vi "zlgcan_demo_USBCANFD_merge.vi"() -> ()   [LabVIEW 2020]
uses:
  zlgcan.lvlib
  data_type/ZCANDataObj.ctl
  data_type/ZCAN_InitCAN_setting_USBCANFD.ctl
  data_type/ZCAN_TransmitFD_frame.ctl
panel:
  in  "canfd_frame":T1
  in  "Clear Data":bool
  in  "stop":bool
  in  "开启CAN":bool
  in  "?":enum32{"DEMO说明", "设备、通道选择", "参数设置", "状态", "发送"}(tab)
  in  "CAN 通道":u32(ring) items=["0", "1"]
  in  "CAN卡型号":u32(ring)=41 items=["USBCANFD-800U"=59, "USBCANFD-200U"=41, "USBCANFD-100U"=42, "USBCANFD-MINI"=43]
  in  "索引":u32(ring) items=["0", "1", "2", "3", "4", "5", "6", "7", "8"]
  out "source":string
  in  "工作模式":u8(ring) items=["正常", "只听"]
  out "can_index_handle(out) 2":u32
  out "Device_handle(out)":u32
  out "can_index_handle(out)":u32
  in  "仲裁域波特率":u32(ring)=500000 items=["1Mbps"=1000000, "800kbps"=800000, "500kbps"=500000, "250kbps"=250000, "125kbps"=125000, "100kbps"=100000, "50kbps"=50000]
  in  "数据域波特率":u32(ring)=500000 items=["5Mbps"=5000000, "4Mbps"=4000000, "2Mbps"=2000000, "1Mbps"=1000000, "800kbps"=800000, "500kbps"=500000, "250kbps"=250000, "125kbps"=125000, "100kbps"=100000]
  in  "自定义波特率字符输入":string
  in  "自定义波特率开关":bool
  out "error out":errorcluster caption="错误输出"
  in  "数据长度":u8=8
  in  "CANFD accelerate":bool
  in  "Chennal":u32
  in  "帧类型":u32(ring) items=["标准帧", "扩展帧"]
  in  "帧格式":u32(ring) items=["数据帧", "远程帧"]
  in  "ID":u32=18 format="0x%08x"
  in  "协议":u32(ring) items=["CAN", "CANFD"]
  in  "数据输入":string="11 22 33 44 55 66 77 88"
  in  "发送":bool
  in  "timeStamp":u64=256
  out "Send Result":bool
  out "CAN报文显示":string[][](table)
  in  "ZCANDataObj":T2[](array[typedef])
  in  "ZCAN_InitCAN_Setting_USBCANFD":T3
  # "1. 确保电脑有VC++ 2005/2008/2010/2013运行库（对应32，64位）,微软常用运行库合集，点击下载（35M）。\n    http://manual.zlg.cn/Public/Uploads/2020-06-05/5ed995c271414.zip"
  # "2，如果打开设备失败，可能原因：\n（1）已经打开过一次，没有正常关闭的情况下，继续点击“打开设备”，是无法打开的。\n     需要USB重新拔插，LABVIEW重启（全部关闭），然后再“打开设备”。\n (2) 项目路径不能有中文繁体。"
  # "适用的设备：USBCANFD-100U、USBCANFD-200U、USBCANFD-MINI、USBCANFD-800U"
  # "停止程序前，\n请先关闭CAN卡"
  # "使用CAN时，\n两个波特率设置相同即可"
  # "使用ZCANPro软件波特率计算工具计算"
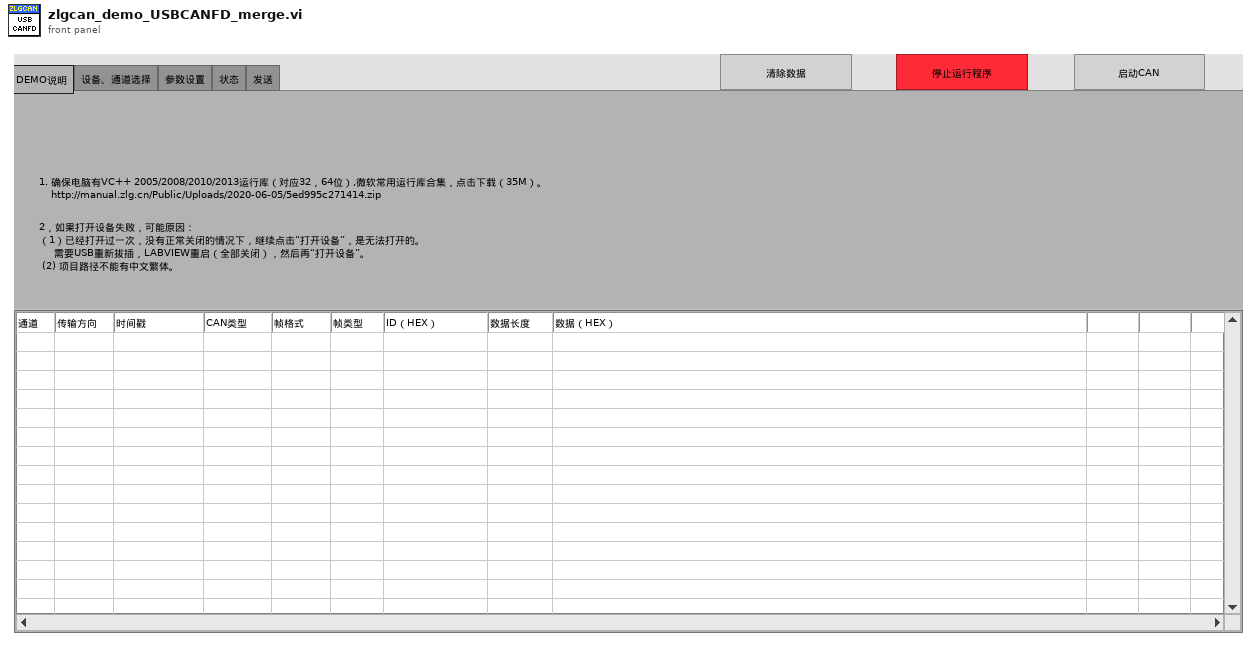
[diagram p1: front panel]
types:
  T1 = typedef "zlgcan.lvlib/ZCAN_TransmitFD_frame.ctl" = cluster{"帧类型":u32, "帧格式":u32, "ID":u32, "数据长度":u8, "CANFD加速？":u8, "DATA":cluster{"CAN数据[0]":u8, "CAN数据[1]":u8, "CAN数据[2]":u8, "CAN数据[3]":u8, "CAN数据[4]":u8, "CAN数据[5]":u8, "CAN数据[6]":u8, "CAN数据[7]":u8, "CAN数据[8]":u8, "CAN数据[9]":u8, "CAN数据[10]":u8, "CAN数据[11] ":u8, "CAN数据[12] ":u8, "CAN数据[13] ":u8, "CAN数据[14] ":u8, "CAN数据[15] ":u8, "CAN数据[16]":u8, "CAN数据[17]":u8, "CAN数据[18]":u8, "CAN数据[19]":u8, "CAN数据[20]":u8, "CAN数据[21]":u8, "CAN数据[22]":u8, "CAN数据[23]":u8, "CAN数据[24] ":u8, "CAN数据[25]":u8, "CAN数据[26]":u8, "CAN数据[27]":u8, "CAN数据[28]":u8, "CAN数据[29]":u8, "CAN数据[30]":u8, "CAN数据[31]":u8, "CAN数据[32]":u8, "CAN数据[33]":u8, "CAN数据[34]":u8, "CAN数据[35]":u8, "CAN数据[36]":u8, "CAN数据[37]":u8, "CAN数据[38]":u8, "CAN数据[39]":u8, "CAN数据[40]":u8, "CAN数据[41]":u8, "CAN数据[42]":u8, "CAN数据[43]":u8, "CAN数据[44]":u8, "CAN数据[45]":u8, "CAN数据[46]":u8, "CAN数据[47]":u8, "CAN数据[48]":u8, "CAN数据[49]":u8, "CAN数据[50]":u8, "CAN数据[51]":u8, "CAN数据[52]":u8, "CAN数据[53]":u8, "CAN数据[54]":u8, "CAN数据[55]":u8, "CAN数据[56]":u8, "CAN数据[57]":u8, "CAN数据[58]":u8, "CAN数据[59]":u8, "CAN数据[60]":u8, "CAN数据[61]":u8, "CAN数据[62]":u8, "CAN数据[63]":u8}}
  T2 = typedef "zlgcan.lvlib/ZCANDataObj.ctl" = cluster{"Data_Type":u8, "CAN_CH":u8, "rawVal(未使用)":u16, "extraData[4]（未使用）":cluster{"[0]":u8, "[1]":u8, "[2]":u8, "[3]":u8}, "canCANFDData":cluster{"时间戳+混合标志位":cluster{"时间戳":u64, "混合标志位":u32}, "extraData[4]（未使用）":cluster{"[0]":u8, "[1]":u8, "[2]":u8, "[3]":u8}, "frame":cluster{"can_id":u32, "Data长度":u8, "CANFD加速？":u8, "__res0":u8, "__res1":u8, "data":cluster{"CANData[0]":u8, "CANData[1]":u8, "CANData[2]":u8, "CANData[3]":u8, "CANData[4]":u8, "CANData[5]":u8, "CANData[6]":u8, "CANData[7]":u8, "CANData[8]":u8, "CANData[9]":u8, "CANData[10]":u8, "CANData[11] ":u8, "CANData[12] ":u8, "CANData[13] ":u8, "CANData[14] ":u8, "CANData[15] ":u8, "CANData[16]":u8, "CANData[17]":u8, "CANData[18]":u8, "CANData[19]":u8, "CANData[20]":u8, "CANData[21]":u8, "CANData[22]":u8, "CANData[23]":u8, "CANData[24] ":u8, "CANData[25]":u8, "CANData[26]":u8, "CANData[27]":u8, "CANData[28]":u8, "CANData[29]":u8, "CANData[30]":u8, "CANData[31]":u8, "CANData[32]":u8, "CANData[33]":u8, "CANData[34]":u8, "CANData[35]":u8, "CANData[36]":u8, "CANData[37]":u8, "CANData[38]":u8, "CANData[39]":u8, "CANData[40]":u8, "CANData[41]":u8, "CANData[42]":u8, "CANData[43]":u8, "CANData[44]":u8, "CANData[45]":u8, "CANData[46]":u8, "CANData[47]":u8, "CANData[48]":u8, "CANData[49]":u8, "CANData[50]":u8, "CANData[51]":u8, "CANData[52]":u8, "CANData[53]":u8, "CANData[54]":u8, "CANData[55]":u8, "CANData[56]":u8, "CANData[57]":u8, "CANData[58]":u8, "CANData[59]":u8, "CANData[60]":u8, "CANData[61]":u8, "CANData[62]":u8, "CANData[63]":u8}}}, "raw":cluster{"[0]":u8, "[1]":u8, "[2]":u8, "[3]":u8, "[4]":u8, "[5]":u8, "[6]":u8, "[7]":u8, "[8]":u8, "[9]":u8, "[10]":u8, "[11]":u8, "[12]":u8, "[13]":u8, "[14]":u8, "[15]":u8, "[16]":u8, "[17]":u8, "[18]":u8, "[19]":u8, "[20]":u8, "[21]":u8, "[22]":u8, "[23]":u8, "[24]":u8, "[25]":u8, "[26]":u8, "[27]":u8, "[28]":u8, "[29]":u8, "[30]":u8, "[31]":u8, "[32]":u8, "[33]":u8, "[34]":u8, "[35]":u8, "[36]":u8, "[37]":u8, "[38]":u8, "[39]":u8, "[40]":u8, "[41]":u8, "[42]":u8, "[43]":u8, "[44]":u8, "[45]":u8, "[46]":u8, "[47]":u8, "[48]":u8, "[49]":u8, "[50]":u8, "[51]":u8, "[52]":u8, "[53]":u8, "[54]":u8, "[55]":u8, "[56]":u8, "[57]":u8, "[58]":u8, "[59]":u8, "[60]":u8, "[61]":u8, "[62]":u8, "[63]":u8, "[64]":u8, "[65]":u8, "[73]":u8, "[72]":u8, "[71]":u8, "[70]":u8, "[69]":u8, "[68]":u8, "[67]":u8, "[66]":u8, "[74]":u8, "[75]":u8, "[83]":u8, "[82]":u8, "[81]":u8, "[80]":u8, "[79]":u8, "[78]":u8, "[77]":u8, "[76]":u8, "[84]":u8, "[85]":u8, "[91]":u8, "[90]":u8, "[89]":u8, "[88]":u8, "[87]":u8, "[86]":u8}}
  T3 = typedef "zlgcan.lvlib/ZCAN_InitCAN_setting_USBCANFD.ctl" = cluster{"abitbaud":u32, "dbitbaud":u32, "baud_rate_custom？":bool, "RateCustom":string, "mode":u8}
  T4 = cluster{"[0]":u32, "[1]":u32, "[2]":u32, "[3]":u32, "[4]":u32, "[5]":u32, "[6]":u32, "[7]":u32, "[8]":u32, "[9]":u32, "[10]":u32, "[11]":u32, "[12]":u32, "[13]":u32, "[14]":u32, "[15]":u32, "[16]":u32, "[17]":u32, "[18]":u32, "[19]":u32, "[20]":u32, "[21]":u32, "[22]":u32, "[23]":u32, "[24]":u32, "[25]":u32, "[26]":u32, "[27]":u32, "[28]":u32, "[29]":u32, "[30]":u32, "[31]":u32, "[32]":u32, "[33]":u32, "[34]":u32, "[35]":u32, "[36]":u32, "[37]":u32, "[38]":u32, "[39]":u32, "[40]":u32, "[41]":u32, "[42]":u32, "[43]":u32, "[44]":u32, "[45]":u32, "[46]":u32, "[47]":u32, "[48]":u32, "[49]":u32, "[50]":u32, "[51]":u32, "[52]":u32, "[53]":u32, "[54]":u32, "[55]":u32, "[56]":u32, "[57]":u32, "[58]":u32, "[59]":u32, "[60]":u32, "[61]":u32, "[62]":u32, "[63]":u32}
  T5 = typedef "ZCANDataObj.ctl" = cluster{"数据类型":u8, "CAN通道号":u8, "rawVal(未使用)":u16, "extraData[4]（未使用）":cluster{"[0]":u8, "[1]":u8, "[2]":u8, "[3]":u8}, "canCANFDData":cluster{"时间戳+混合标志位":cluster{"时间戳":u64, "混合标志位":u32}, "extraData[4]（未使用）":cluster{"[0]":u8, "[1]":u8, "[2]":u8, "[3]":u8}, "frame":cluster{"can_id":u32, "数据长度":u8, "CANFD加速？":u8, "__res0":u8, "__res1":u8, "data":cluster{"CAN数据[0]":u8, "CAN数据[1]":u8, "CAN数据[2]":u8, "CAN数据[3]":u8, "CAN数据[4]":u8, "CAN数据[5]":u8, "CAN数据[6]":u8, "CAN数据[7]":u8, "CAN数据[8]":u8, "CAN数据[9]":u8, "CAN数据[10]":u8, "CAN数据[11] ":u8, "CAN数据[12] ":u8, "CAN数据[13] ":u8, "CAN数据[14] ":u8, "CAN数据[15] ":u8, "CAN数据[16]":u8, "CAN数据[17]":u8, "CAN数据[18]":u8, "CAN数据[19]":u8, "CAN数据[20]":u8, "CAN数据[21]":u8, "CAN数据[22]":u8, "CAN数据[23]":u8, "CAN数据[24] ":u8, "CAN数据[25]":u8, "CAN数据[26]":u8, "CAN数据[27]":u8, "CAN数据[28]":u8, "CAN数据[29]":u8, "CAN数据[30]":u8, "CAN数据[31]":u8, "CAN数据[32]":u8, "CAN数据[33]":u8, "CAN数据[34]":u8, "CAN数据[35]":u8, "CAN数据[36]":u8, "CAN数据[37]":u8, "CAN数据[38]":u8, "CAN数据[39]":u8, "CAN数据[40]":u8, "CAN数据[41]":u8, "CAN数据[42]":u8, "CAN数据[43]":u8, "CAN数据[44]":u8, "CAN数据[45]":u8, "CAN数据[46]":u8, "CAN数据[47]":u8, "CAN数据[48]":u8, "CAN数据[49]":u8, "CAN数据[50]":u8, "CAN数据[51]":u8, "CAN数据[52]":u8, "CAN数据[53]":u8, "CAN数据[54]":u8, "CAN数据[55]":u8, "CAN数据[56]":u8, "CAN数据[57]":u8, "CAN数据[58]":u8, "CAN数据[59]":u8, "CAN数据[60]":u8, "CAN数据[61]":u8, "CAN数据[62]":u8, "CAN数据[63]":u8}}}, "Reserve":u32}
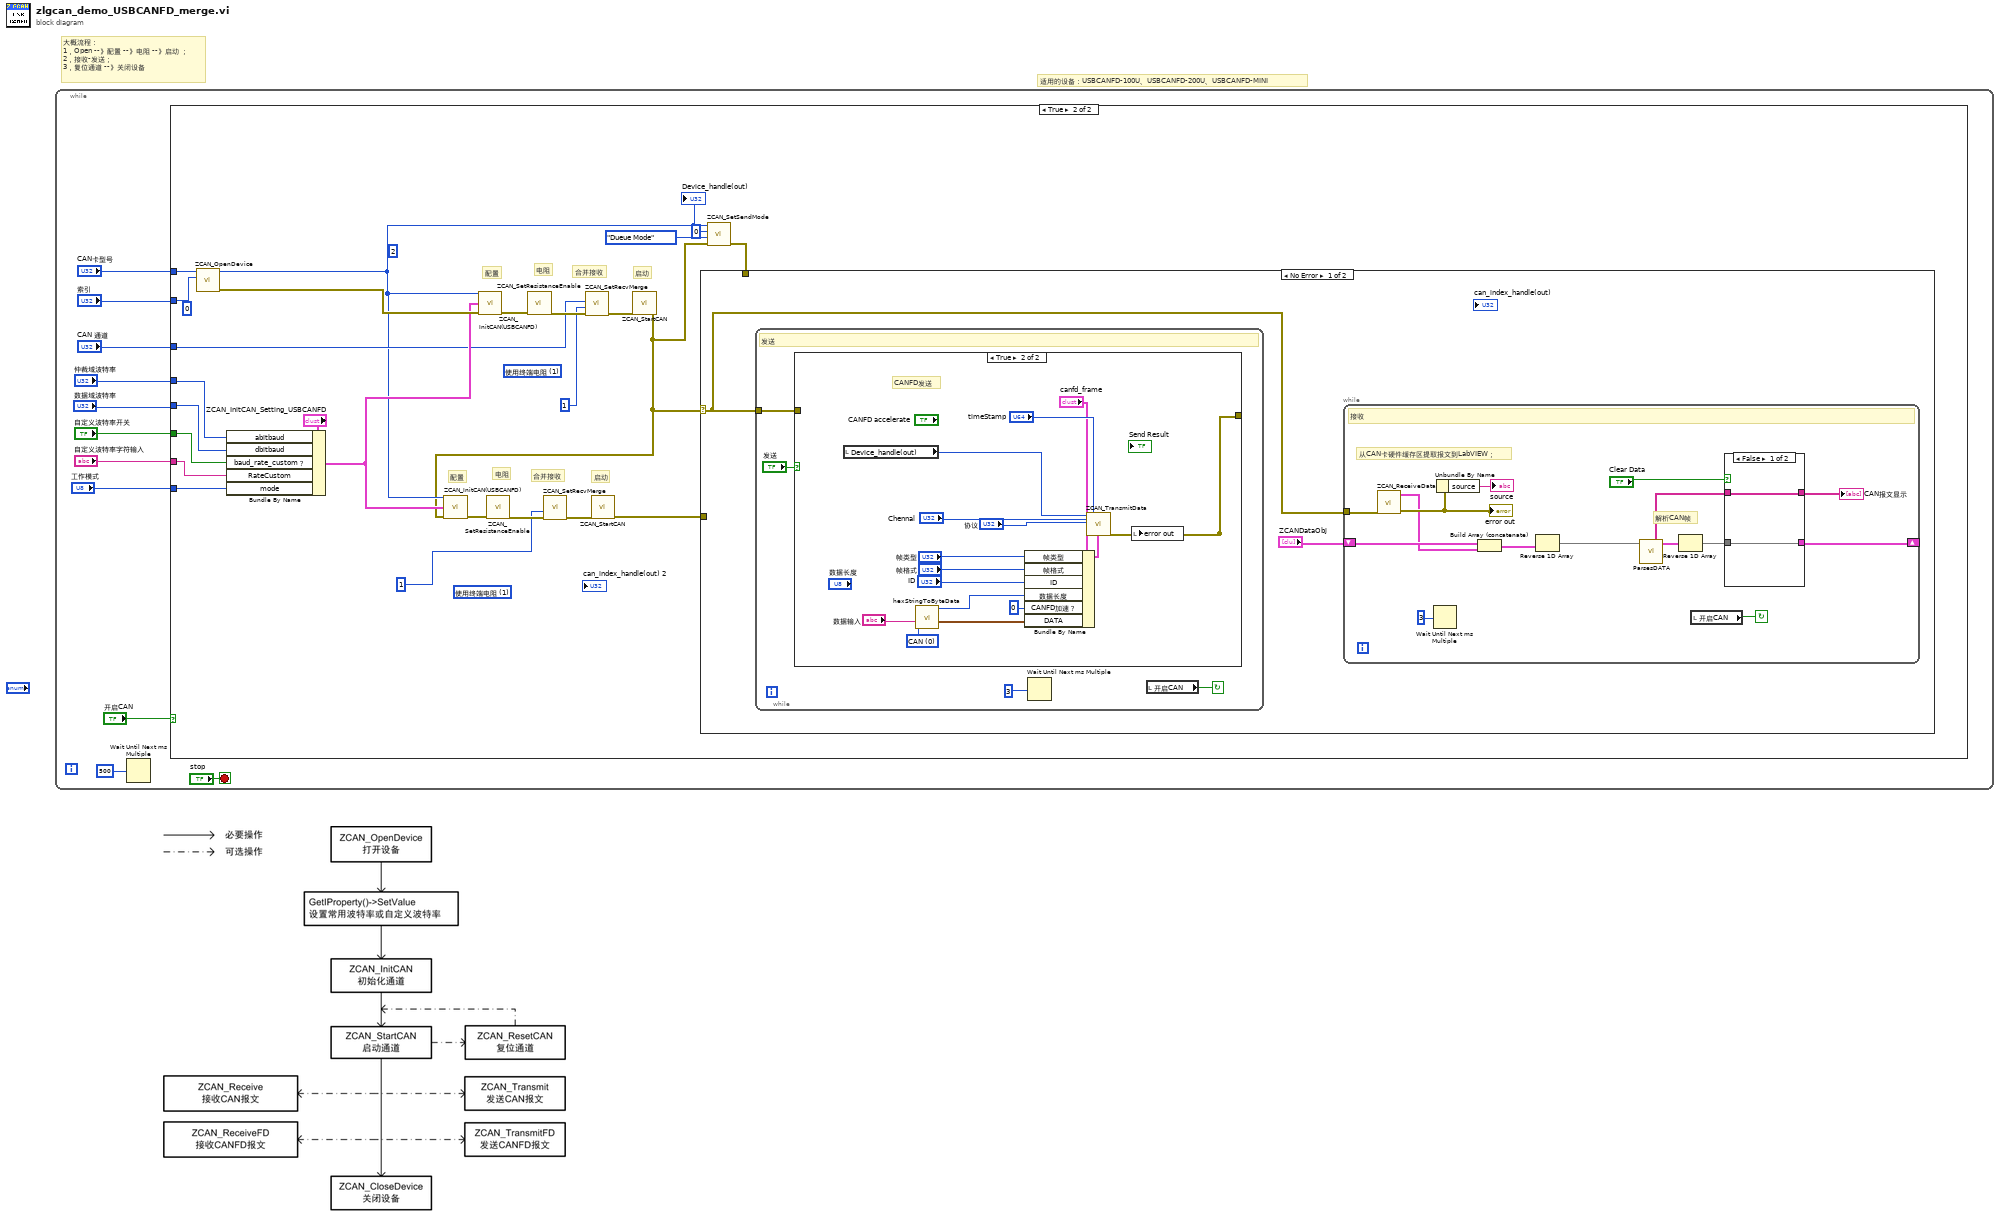
[diagram p0: block diagram]
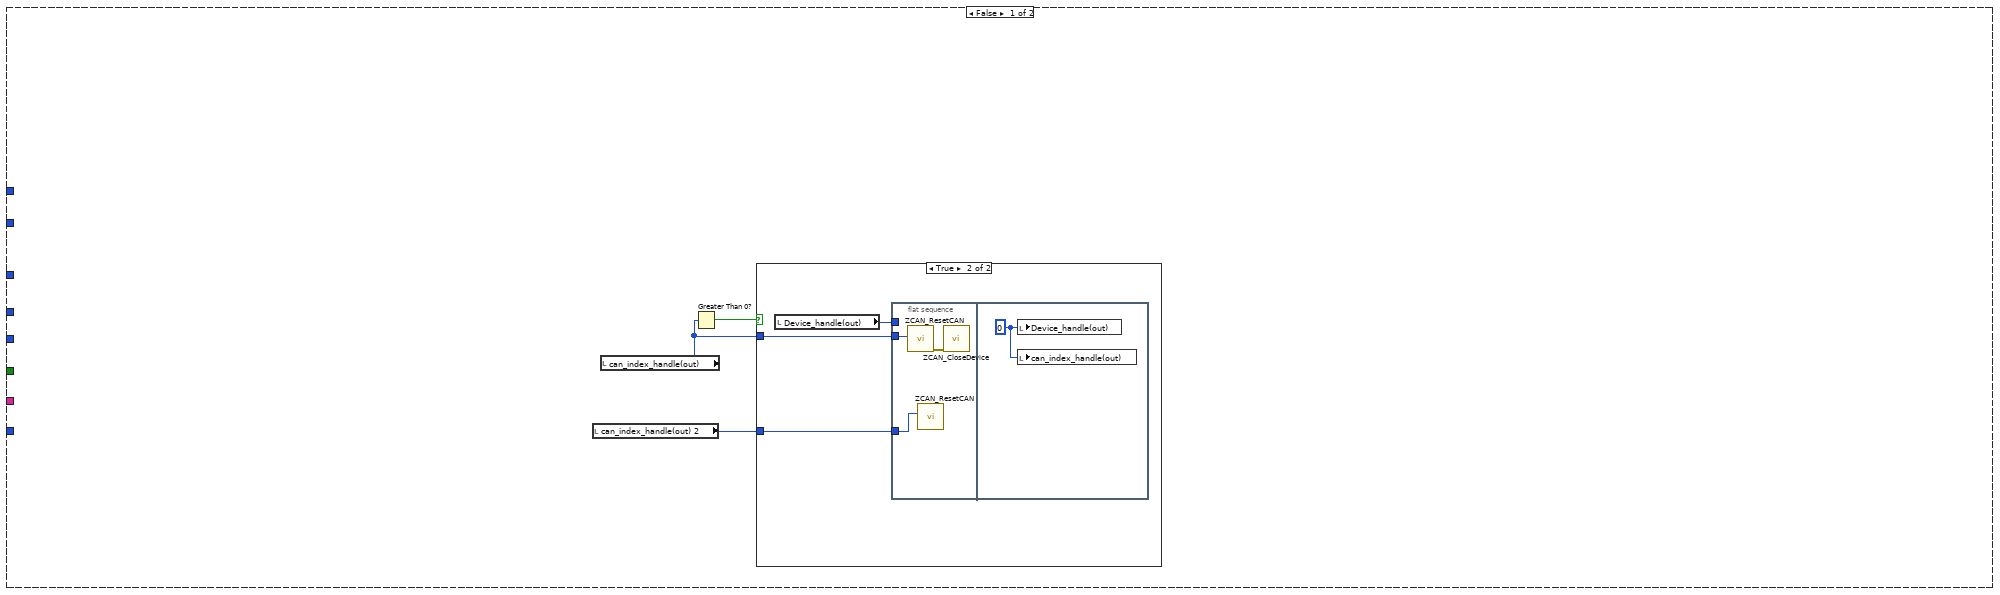
[diagram p2: hidden frame]
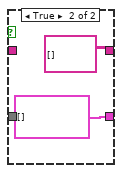
[diagram p4: hidden frame]
diagram:
  # "大概流程：\n1，Open --》配置 --》电阻 --》启动 ；\n2，接收-发送；\n3，复位通道 --》关闭设备"
  # "适用的设备：USBCANFD-100U、USBCANFD-200U、USBCANFD-MINI"
  n1 = while {
    stop <- "stop" stop-if-true
    n2 = Wait Until Next ms Multiple(millisecond multiple=u32 500) -> ()  [unwired: 1 out]
    n3 = case shown="True" "开启CAN" {
      tunnel: "CAN 通道" -> [_ w28]
      tunnel: "仲裁域波特率" -> [_ w41]
      tunnel: "自定义波特率开关" -> [_ w43]
      tunnel: "自定义波特率字符输入" -> [_ w40]
      tunnel: "工作模式" -> [_ w39]
      tunnel: "CAN卡型号" -> [_ w45]
      tunnel: "索引" -> [_ w46]
      tunnel: "数据域波特率" -> [_ w42]
      frame False {
        # "关闭CAN卡"
        n4 = local read "can_index_handle(out) 2"() -> (w12:u32)
        n5 = local read "can_index_handle(out)"() -> (w13:u32)
        n6 = Greater Than 0?(x=w13) -> (x > 0?=w14:bool)
        n7 = case shown="True" w14 {
          tunnel: w13 -> [_ w17]
          tunnel: w12 -> [_ w15]
          frame False {
          }
          frame True {
            n8 = local read "Device_handle(out)"() -> (w16:u32)
            n9 = flat-sequence {
              tunnel: w17 -> [w19]
              tunnel: w16 -> [_]
              tunnel: w15 -> [w18]
              frame #0 {
                n10 = call "ZCAN_ResetCAN.vi"(10:w19) -> ("error out"=w20:errorcluster)  [unwired: 10 in]
                n11 = call "ZCAN_ResetCAN.vi"(10:w18) -> ()  [unwired: 10 in, 1 out]
                n12 = call "ZCAN_CloseDevice.vi"("error in (no error)"=w20) -> ()  [unwired: 10 in, 1 out]
              }
              frame #1 {
                w21 = u32 0 ("can_index_handle(out)")
                n13 = local write "Device_handle(out)"(w21) -> ()
                n14 = local write "can_index_handle(out)"(w21) -> ()
              }
            }
          }
        }
      }
      frame True {
        (unwired) u8 1 items=["不使用终端电阻", "使用终端电阻"] ("是否使用电阻")
        (unwired) u8 1 items=["不使用终端电阻", "使用终端电阻"] ("是否使用电阻")
        (unwired) 2
        (unwired) 0
        # "合并接收"
        # "启动"
        # "电阻"
        # "配置"
        # "合并接收"
        # "启动"
        # "电阻"
        # "配置"
        n15 = call "ZCAN_OpenDevice.vi"("device_index"=w46, "device_type"=w45) -> ("error out"=w38:errorcluster, "DEVICE_HANDLE"=w26:u32)  [unwired: 6 in, 2 out]
        "Device_handle(out)" <- w26
        n16 = Bundle By Name(cluster="ZCAN_InitCAN_Setting_USBCANFD", "abitbaud"=w41, "dbitbaud"=w42, "baud_rate_custom？"=w43, "RateCustom"=w40, "mode"=w39) -> (w30:T3)
        n17 = call "ZCAN_InitCAN(USBCANFD).vi"("device_hande"=w26, "ZCAN_InitCAN_Setting_USBCANFD"=w30, "error in (no error)"=w38) -> ("error out"=w37:errorcluster)  [unwired: 11 in, 1 out]
        n18 = call "ZCAN_SetResistanceEnable.vi"("error in (no error)"=w37) -> ("error out"=w35:errorcluster)  [unwired: 9 in, 1 out]
        n19 = call "ZCAN_SetRecvMerge.vi"("Enable"=w28, "can通道"=1 ("Enable"), "error in (no error)"=w35) -> ("error out"=w36:errorcluster)  [unwired: 6 in, 1 out]
        n20 = call "ZCAN_StartCAN.vi"("error in (no error)"=w36) -> ("error out"=w22:errorcluster)  [unwired: 9 in, 1 out]
        n21 = call "ZCAN_InitCAN(USBCANFD).vi"("device_hande"=w26, "ZCAN_InitCAN_Setting_USBCANFD"=w30, "error in (no error)"=w22) -> ("error out"=w32:errorcluster)  [unwired: 11 in, 1 out]
        n22 = call "ZCAN_SetResistanceEnable.vi"("error in (no error)"=w32) -> ("error out"=w34:errorcluster)  [unwired: 9 in, 1 out]
        n23 = call "ZCAN_SetRecvMerge.vi"("can通道"=1, "error in (no error)"=w34) -> ("error out"=w33:errorcluster)  [unwired: 7 in, 1 out]
        n24 = call "ZCAN_StartCAN.vi"("error in (no error)"=w33) -> ("error out"=w29:errorcluster)  [unwired: 9 in, 1 out]
        n25 = call "ZCAN_SetSendMode.vi"("error in (no error)"=w22, "SendMode"=enum16{"Normal Mode", "Dueue Mode"}."Dueue Mode", "CH_ID"=0, "DeviceHANDLE"=w26) -> ("error out"=w23:errorcluster)  [unwired: 7 in]
        n26 = case shown="No Error" w22 {
          selector: w22 -> [w48 _]
          tunnel: w29 -> [_ _]
          tunnel: w23 -> [_ _]
          frame No Error {
            n27 = while {
              tunnel: w48 -> [w68]
              stop <- w69 continue-if-true
              # "发送"
              n28 = case shown="True" "发送" {
                tunnel: w68 -> [w72 _]
                tunnel: [w72 w87] -> _
                frame False {
                }
                frame True {
                  w76 = u32 0 items=["CAN", "CANFD"] ("协议")
                  # "CANFD发送"
                  n29 = local read "Device_handle(out)"() -> (w85:u32)
                  n30 = call "hexStringToByteData.vi"("数据输入"="数据输入", "协议"=w76) -> ("CANFD_data"=w75:T4, "字节数"=w73:u8)  [unwired: 6 in, 2 out]
                  n31 = Bundle By Name(cluster="canfd_frame", "帧类型"="帧类型", "帧格式"="帧格式", "ID"="ID", "数据长度"=w73, "CANFD加速？"=u8 0, "DATA"=w75) -> (w81:T1)
                  n32 = call "ZCAN_TransmitData.vi"("can_index_handle"=w85, "CAN通道号"="Chennal", "协议"="协议", "timeStamp"="timeStamp", "canfd_frame"=w81) -> ("error out"=w87:errorcluster)  [unwired: 14 in]
                  n33 = local write "error out"(w87) -> ()
                }
              }
              n34 = Wait Until Next ms Multiple(millisecond multiple=u32 3) -> ()  [unwired: 1 out]
              n35 = local read "开启CAN"() -> (w69:bool)
            }
            n36 = while {
              tunnel: w48 -> [w62]
              shift-right: [w50] -> _
              shift-left: "ZCANDataObj" -> [w60]
              stop <- w61 continue-if-true
              # "从CAN卡硬件缓存区提取报文到LabVIEW；"
              # "解析CAN帧"
              # "接收"
              n37 = call "ZCAN_ReceiveData.vi"("error in (no error)"=w62) -> ("error out"=w57:errorcluster, "ZCANDataObj（out）"=w56:T2[])  [unwired: 3 in, 1 out]
              "error out" <- w57
              n38 = Wait Until Next ms Multiple(millisecond multiple=u32 3) -> ()  [unwired: 1 out]
              n39 = Unbundle By Name(w57) -> ("source"=→"source":string)
              n40 = Build Array (concatenate)(w60, w56) -> (w59:T2[])
              n41 = Reverse 1D Array(array=w59) -> (reversed array=w55:T2[])
              n42 = call "ParsesDATA.vi"("ZCANDataObj"=w55) -> ("ZCANDataObj(out)"=w54:T5[], "CAN报文显示"=w51:string[][])  [unwired: 9 in]
              n43 = Reverse 1D Array(array=w54) -> (reversed array=w49:T5[])
              n44 = local read "开启CAN"() -> (w61:bool)
              n45 = case shown="False" "Clear Data" {
                tunnel: w51 -> [w65 _]
                tunnel: [w65 string[][] [] ("CAN报文显示")] -> w53
                tunnel: [w64 T2[] [] ("Array")] -> w50
                tunnel: w49 -> [w64 _]
                frame False {
                }
                frame True {
                }
              }
              "CAN报文显示" <- w53
            }
          }
          frame Error {
          }
        }
      }
    }
  }
